vi "Plotter_UI_Plot.vi"(8 "error in (no error)":errorcluster, 11 "Globals":T1) -> ()   [LabVIEW 2017]
uses:
  Controls/Plotter_Globals.ctl
  Classes/ADCP.lvclass
  Controls/Plotter_Queues.ctl
  Controls/Plotter_Queue_Command_and_Data.ctl
  Controls/Plotter_Commands.ctl
  Controls/Plotter_Plot_Parameter_and_Timestamp.ctl
  Controls/Plotter_UI_Plot_Commands.ctl
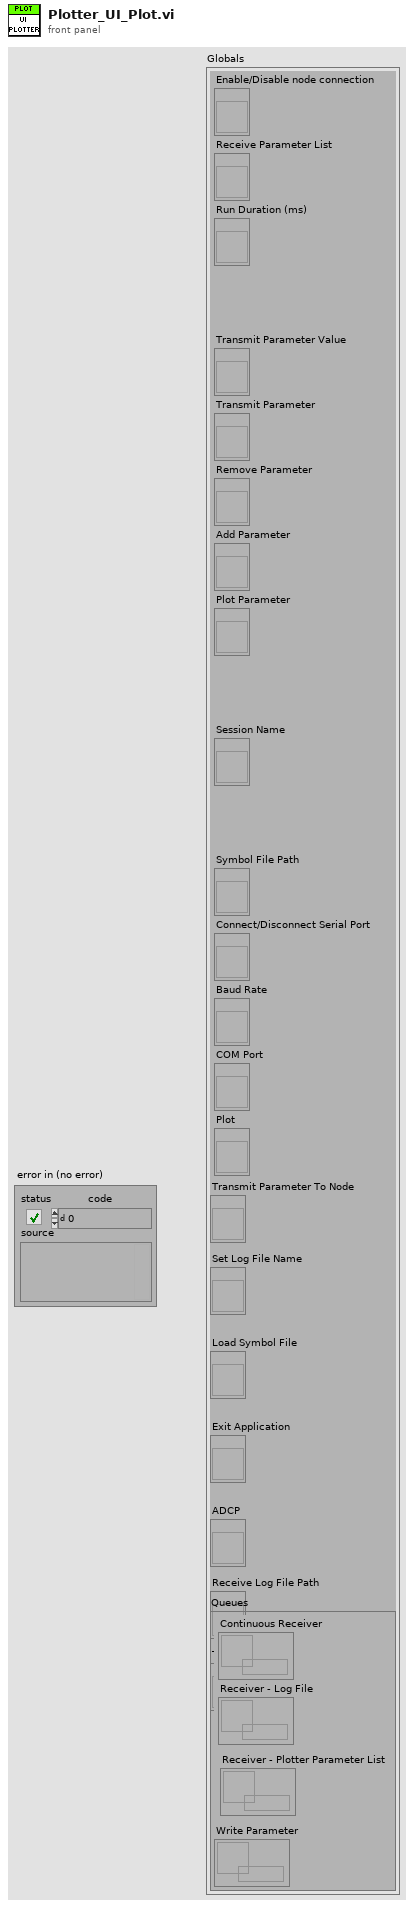
[diagram p1: front panel]
types:
  T1 = typedef "Plotter_Globals.ctl" = cluster{"Enable/Disable node connection":refnum<vi>, "Receive Parameter List":refnum<vi>, "Run Duration (ms)":refnum<vi>, "Transmit Parameter Value":refnum<vi>, "Transmit Parameter":refnum<vi>, "Remove Parameter":refnum<vi>, "Add Parameter":refnum<vi>, "Plot Parameter":refnum<vi>, "Session Name":refnum<vi>, "Symbol File Path":refnum<vi>, "Connect/Disconnect Serial Port":refnum<vi>, "Baud Rate":refnum<vi>, "COM Port":refnum<vi>, "Plot":refnum<vi>, "Transmit Parameter To Node":refnum<vi>, "Set Log File Name":refnum<vi>, "Load Symbol File":refnum<vi>, "Exit Application":refnum<vi>, "ADCP":refnum<vi>, "Transmit Log File Path":refnum<vi>, "Receive Log File Path":refnum<vi>, "Queues":T2}
  T2 = typedef "Plotter_Queues.ctl" = cluster{"Continuous Receiver":refnum<queue>, "Receiver - Log File":refnum<queue>, "Receiver - Plotter Parameter List":refnum<queue>, "Write Parameter":refnum<queue>}
  T3 = typedef "Plotter_Commands.ctl" = enum16{"Idle", "Cont_RX_Open_Node", "Cont_RX_Flush_Serial_Port", "Cont_Rx_Log_Write", "Plot_Update", "Exit"}
  T4 = typedef "Plotter_UI_Plot_Commands.ctl" = enum16{"Initialize", "Update", "Clear"}
  T5 = typedef "Plotter_Plot_Parameter_and_Timestamp.ctl" = cluster{"Parameter":string, "Value":string, "Time (ms)":u32}
  T6 = typedef "Plotter_Queue_Command_and_Data.ctl" = cluster{"Commands":T3, "Data":variant}
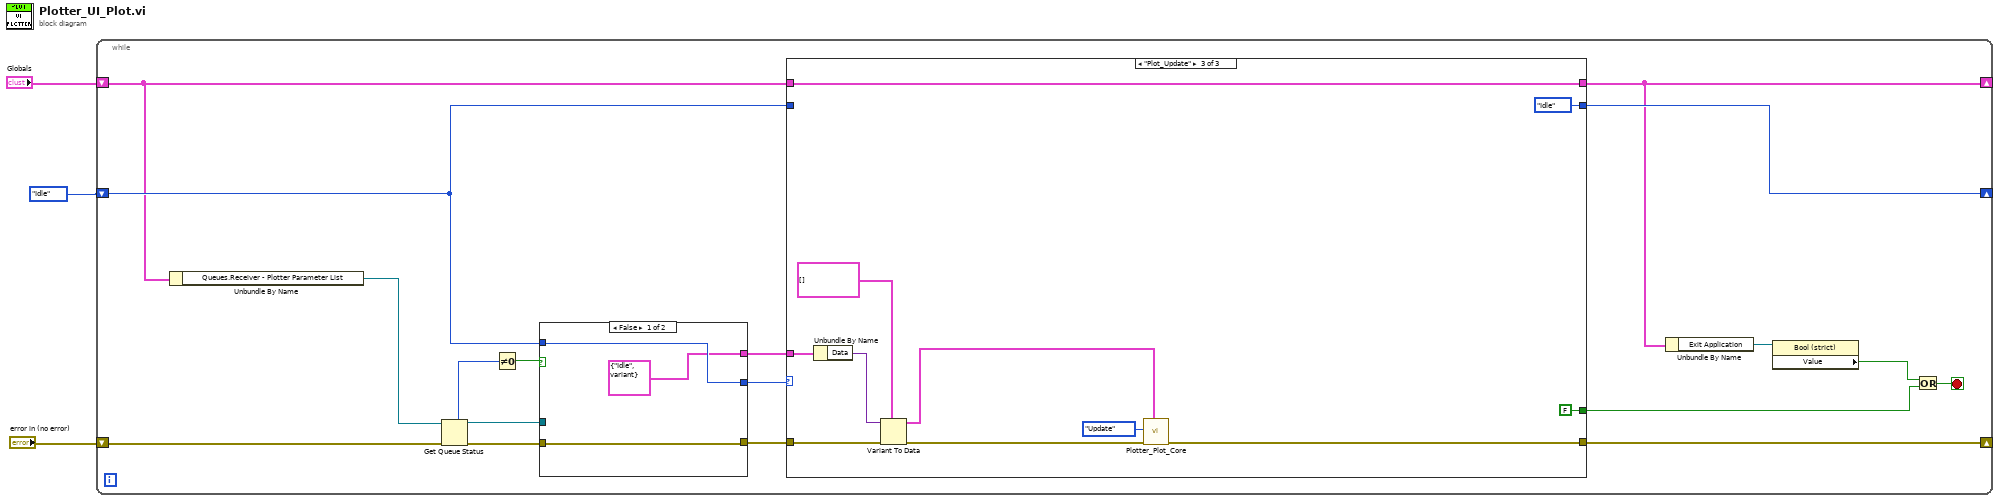
[diagram p0: block diagram]
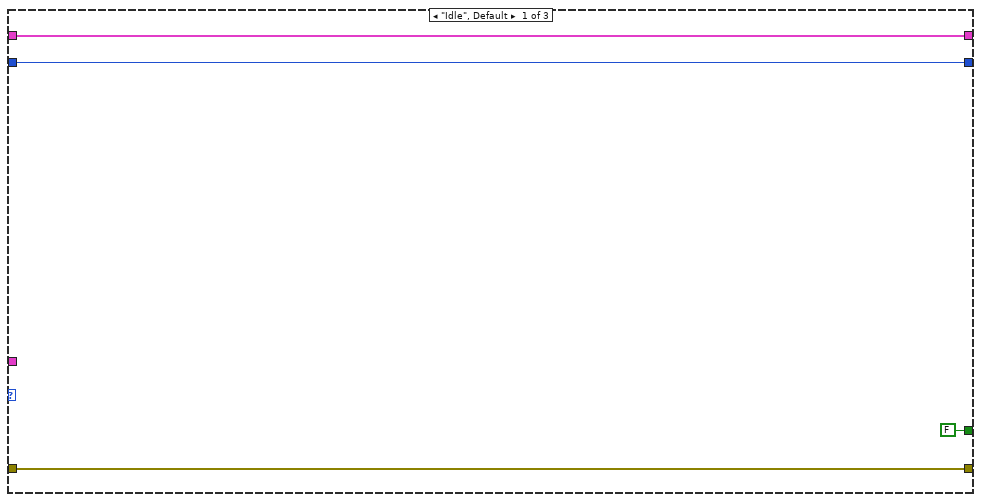
[diagram p2: hidden frame]
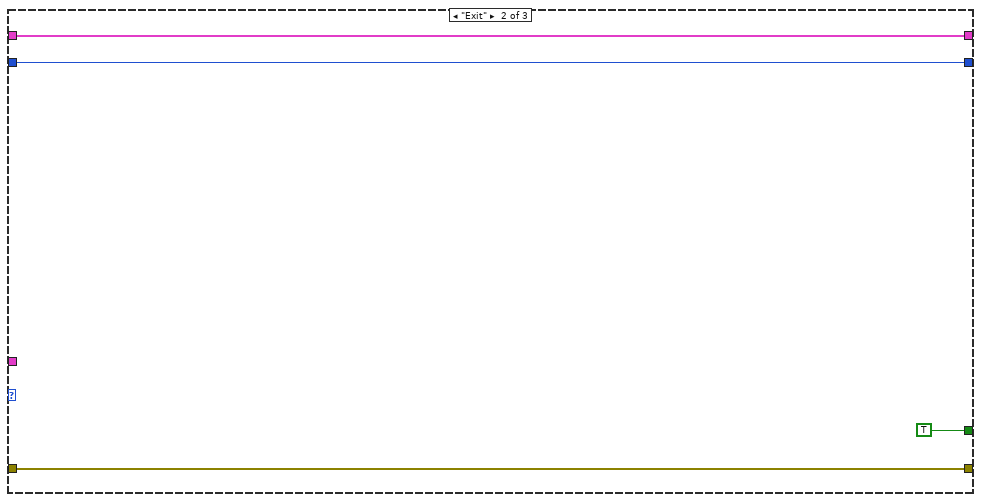
[diagram p3: hidden frame]
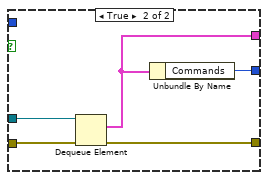
[diagram p4: hidden frame]
diagram:
  n1 = while {
    shift-right: [w13] -> _
    shift-left: "error in (no error)" -> [w21]
    shift-right: [w7] -> _
    shift-left: "Globals" -> [w11]
    shift-right: [w10] -> _
    shift-left: Plotter_Commands."Idle" ("Commands") -> [w12]
    stop <- w9 stop-if-true
    n2 = Unbundle By Name(w11) -> ("Queues.Receiver - Plotter Parameter List"=w20:refnum<queue>)
    n3 = Get Queue Status(queue=w20, error in (no error)=w21) -> (queue out=w16:refnum<queue>, error out=w17:errorcluster, # elements in queue=w19:i32)  [unwired: 1 in, 5 out]
    n4 = Not Equal To 0?(x=w19) -> (x != 0?=w18:bool)
    n5 = case shown="False" w18 {
      tunnel: w17 -> [w42 w48]
      tunnel: w16 -> [_ w47]
      tunnel: [w42 w46] -> w14
      tunnel: [w43 w45] -> w15
      tunnel: w12 -> [w43 _]
      tunnel: [T6 {"Commands"=enum."Idle", "Data"=variant} ("Plotter_Queue_Command_and_Data") w44] -> w4
      frame False {
      }
      frame True {
        n6 = Dequeue Element(queue=w47, error in (no error)=w48) -> (element=w44:T6, error out=w46:errorcluster)  [unwired: 1 in, 2 out]
        n7 = Unbundle By Name(w44) -> ("Commands"=w45:T3)
      }
    }
    n8 = case shown="\"Plot_Update\"" w15 {
      tunnel: w14 -> [w25 w29 w35]
      tunnel: [w25 w29 w38] -> w13
      tunnel: [FALSE TRUE FALSE] -> w8
      tunnel: w12 -> [w22 w26 _]
      tunnel: w11 -> [w23 w27 w40]
      tunnel: [w23 w27 w40] -> w7
      tunnel: [w22 w26 Plotter_Commands."Idle" ("Commands")] -> w10
      tunnel: w4 -> [_ _ w36]
      frame "Idle", Default {
      }
      frame "Exit" {
      }
      frame "Plot_Update" {
        n9 = Unbundle By Name(w36) -> ("Data"=w33:variant)
        n10 = Variant To Data(error in=w35, type=T5[] [], Variant=w33) -> (data=w31:T5[], error out=w34:errorcluster)
        n11 = call "Plotter_Plot_Core.vi"("Plot Parameters"=w31, "error in (no error)"=w34, "Commands"=Plotter_UI_Plot_Commands."Update") -> ("error out"=w38:errorcluster)  [unwired: 8 in]
      }
    }
    n12 = Unbundle By Name(w7) -> ("Exit Application"=w6:refnum<vi>)
    n13 = property class="Bool (strict)"(reference=w6) -> ("Value"=w5:bool)  [unwired: 1 in, 2 out]
    n14 = Or(x=w5, y=w8) -> (x .or. y?=w9:bool)
  }
